vi "Translator.FormatMessage.vi"(8 "error in (no error)":errorcluster, 9 "Arguments":variant[](array[variant]), 10 "Msg":string) -> (0 "error out":errorcluster, 2 "Translated Msg":string)   [LabVIEW 2019, in "Tools.lvlib"]
uses:
  Tools.lvlib
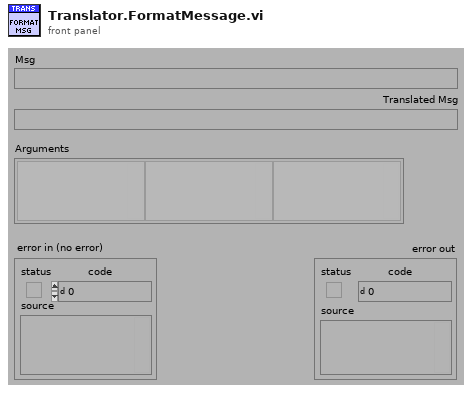
[diagram p1: front panel]
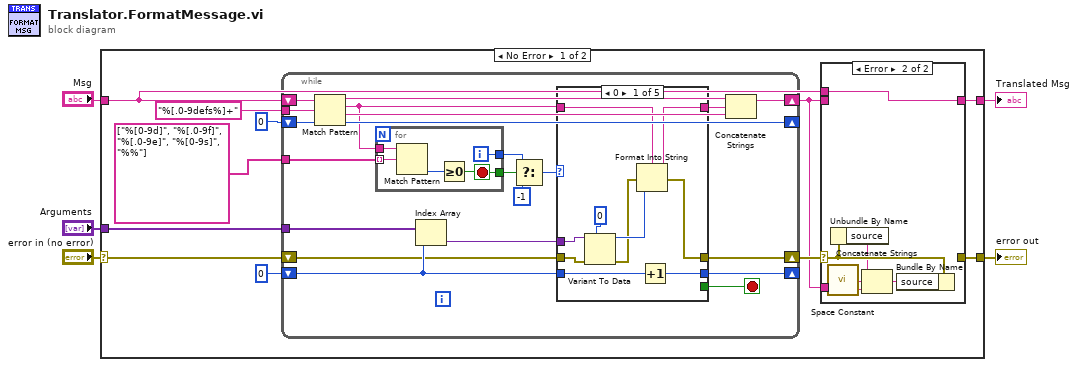
[diagram p0: block diagram]
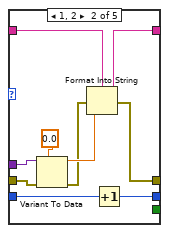
[diagram p3: hidden frame]
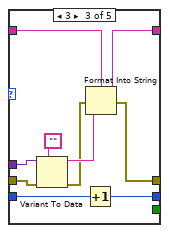
[diagram p4: hidden frame]
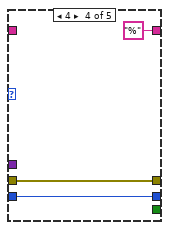
[diagram p5: hidden frame]
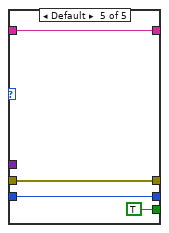
[diagram p6: hidden frame]
diagram:
  n1 = case shown="No Error" "error in (no error)" {
    selector: "error in (no error)" -> [w13 w88]
    tunnel: "Msg" -> [w6 w89]
    tunnel: "Arguments" -> [w14 _]
    tunnel: [w7 w89] -> w3
    tunnel: [w9 w88] -> w1
    frame No Error {
      n2 = while {
        tunnel: string[] ["%[0-9d]", "%[.0-9f]", "%[.0-9e]", "%[0-9s]", "%%"] -> [w41]
        shift-right: [w45] -> _
        shift-left: 0 -> [w43]
        shift-right: [w33] -> _
        shift-left: 0 -> [w34]
        tunnel: w14 -> [w44]
        shift-right: [w25] -> w8
        shift-left: w6 -> [w36]
        shift-right: [w38] -> w10
        shift-left: w13 -> [w39]
        tunnel: "%[.0-9defs%]+" -> [w35]
        stop <- w40 stop-if-true
        n3 = Match Pattern(string=w36, regular expression=w35, offset (0)=w34) -> (before substring=w28:string, match substring=w26:string, after substring=w27:string, offset past match=w33:i32)
        n4 = for {
          tunnel: w26 -> [w87]
          tunnel: w41 -> [w86] mode=indexing
          tunnel: [w83] -> w30
          tunnel: [w84] -> w32
          i -> [w83]
          stop <- w84 stop-if-true
          n5 = Match Pattern(string=w87, regular expression=w86) -> (offset past match=w85:i32)  [unwired: 1 in, 3 out]
          n6 = Greater Or Equal To 0?(x=w85) -> (x >= 0?=w84:bool)
        }
        n7 = Index Array(array=w44, index=w43) -> (element=w42:variant)
        n8 = Select(t=w30, s=w32, f=-1) -> (s? t:f=w31:i32)
        n9 = case shown="0" w31 {
          tunnel: w43 -> [w52 w62 w73 w76 w82]
          tunnel: [w55 w65 w75 w76 w82] -> w45
          tunnel: w26 -> [w54 w64 w74 _ w79]
          tunnel: w42 -> [w50 w60 w71 _ _]
          tunnel: [w46 w56 w66 "%" ("Msg") w79] -> w37
          tunnel: [_ _ _ _ TRUE] -> w40
          tunnel: w39 -> [w49 w59 w69 w77 w80]
          tunnel: [w47 w57 w67 w77 w80] -> w38
          frame 0 {
            n10 = Variant To Data(error in=w49, type=0, Variant=w50) -> (data=w51:i32, error out=w48:errorcluster)
            n11 = Format Into String(format string=w54, error in=w48, w51) -> (resulting string=w46:string, error out=w47:errorcluster)  [unwired: 1 in]
            n12 = Increment(x=w52) -> (x+1=w55:i32)
          }
          frame 1, 2 {
            n13 = Variant To Data(error in=w59, type=0.0, Variant=w60) -> (data=w61:dbl, error out=w58:errorcluster)
            n14 = Format Into String(format string=w64, error in=w58, w61) -> (resulting string=w56:string, error out=w57:errorcluster)  [unwired: 1 in]
            n15 = Increment(x=w62) -> (x+1=w65:i32)
          }
          frame 3 {
            n16 = Variant To Data(error in=w69, type="", Variant=w71) -> (data=w72:string, error out=w68:errorcluster)
            n17 = Increment(x=w73) -> (x+1=w75:i32)
            n18 = Format Into String(format string=w74, error in=w68, w72) -> (resulting string=w66:string, error out=w67:errorcluster)  [unwired: 1 in]
          }
          frame 4 {
          }
          frame Default {
          }
        }
        n19 = Concatenate Strings(w28, w37, w27) -> (w25:string)
      }
      n20 = case shown="Error" w10 {
        selector: w10 -> [w18 w23]
        tunnel: [w18 _] -> w9
        tunnel: w8 -> [_ w21]
        tunnel: w8 -> [w17 _]
        tunnel: [w17 w19] -> w7
        tunnel: w6 -> [_ w19]
        frame No Error {
        }
        frame Error {
          n21 = call <vilib>:"Space Constant.vi"() -> ("String"=w20:string)
          n22 = Unbundle By Name(w23) -> ("source"=w22:string)
          n23 = Concatenate Strings(w22, w20, w21) -> (w24:string)
          n24 = Bundle By Name(cluster=w23, "source"=w24) -> ()  [unwired: 1 out]
        }
      }
    }
    frame Error {
    }
  }
  "Translated Msg" <- w3
  "error out" <- w1
